vi "Peak.vi"(11 "POTTypedCircularBuffer in":refnum<class "POTTypedCircularBuffer.lvclass">) -> (2 "element":T1, 3 "POTTypedCircularBuffer out":refnum<class "POTTypedCircularBuffer.lvclass">)   [LabVIEW 2024, in "POTTypedCircularBuffer.lvclass"]
uses:
  POTTypedCircularBuffer.lvclass
  POTTypedCircularBuffer.lvclass/POTTypedCircularBuffer.ctl
  Type.ctl
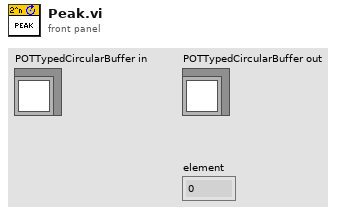
[diagram p1: front panel]
types:
  T1 = typedef "POTTypedCircularBuffer.lvclass/Type.ctl" = i32
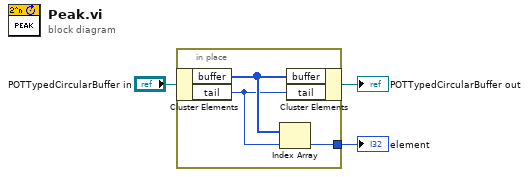
[diagram p0: block diagram]
diagram:
  n1 = in-place {
    in-place-border: [w5] -> w1
    n2 = in-place-cluster #1("POTTypedCircularBuffer in") -> ("buffer"=w6:T1[], "tail"=w4:i32)
    n3 = Index Array(array=w6, index=w4) -> (element=w5:T1)
    n4 = in-place-cluster #1("buffer"=w6, "tail"=w4) -> (→"POTTypedCircularBuffer out":refnum<class "POTTypedCircularBuffer.lvclass">)
  }
  "element" <- w1
